vi "Initialise.vi"(8 "error in (no error)":errorcluster, 10 "Message in":refnum<class "InitialiseMessage.lvclass">, 11 "StageSPIM in":refnum<class "StageSPIM.lvclass">) -> (0 "error out":errorcluster, 3 "StageSPIM out":refnum<class "StageSPIM.lvclass">)   [LabVIEW 2012, in "StageSPIM.lvclass"]
doc: "This method is called when an initialise message is received. It mainly initialises the RabbitMQ connectivity. \n\nOverride this method when your component needs special initialisation (e.g. of software or hardware resources). In that case, don't forget to call the parent for proper implementation. If your component owns subcomponents, they count as resources, so you have to initialise them by calling their own initialise functions"
uses:
  StageSPIM.lvclass
  <vilib>/Distrio/Murmex/InitialiseMessage/InitialiseMessage.lvclass
  <vilib>/Distrio/Murmex/Murmex/Murmex.lvclass
  StageSPIM.lvclass/StageSPIM.ctl
panel:
  # "This method is called when the INTIALISE\ntrigger is sent. \n\nOverride this method when your component needs to\nrespond to this trigger. \n\nCall parent for proper implementation"
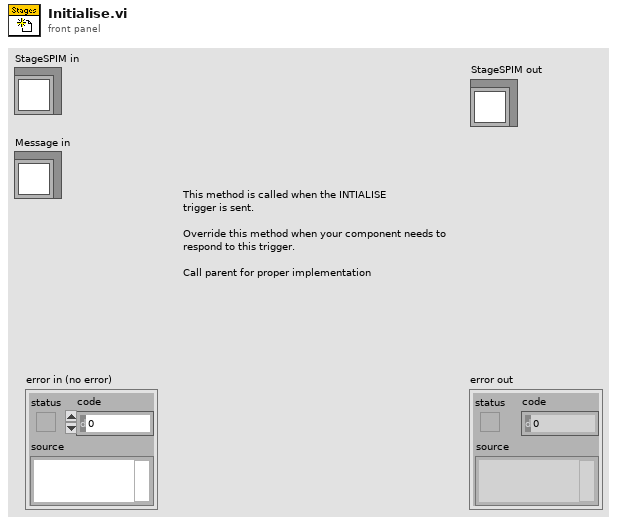
[diagram p1: front panel]
types:
  T1 = cluster{"Register DC":bool, "DaisyChain Search?":bool, "Device ID":i32}[][]
  T2 = cluster{"RON Affected axes":string[], "Reference mode":bool[], "Check FRF?":bool}
  T3 = typedef "StageSPIM.lvclass/port_control.ctl" = i32
  T4 = typedef "StageSPIM.lvclass/baud_rate_control.ctl" = u16
  T5 = typedef "StageSPIM.lvclass/connection_type.ctl" = enum16{"RS232", "RS232 DaisyChain", "USB", "USB_DaisyChain"}
  T6 = cluster{"Register DC":bool, "DaisyChain Search?":bool, "Device ID":i32}
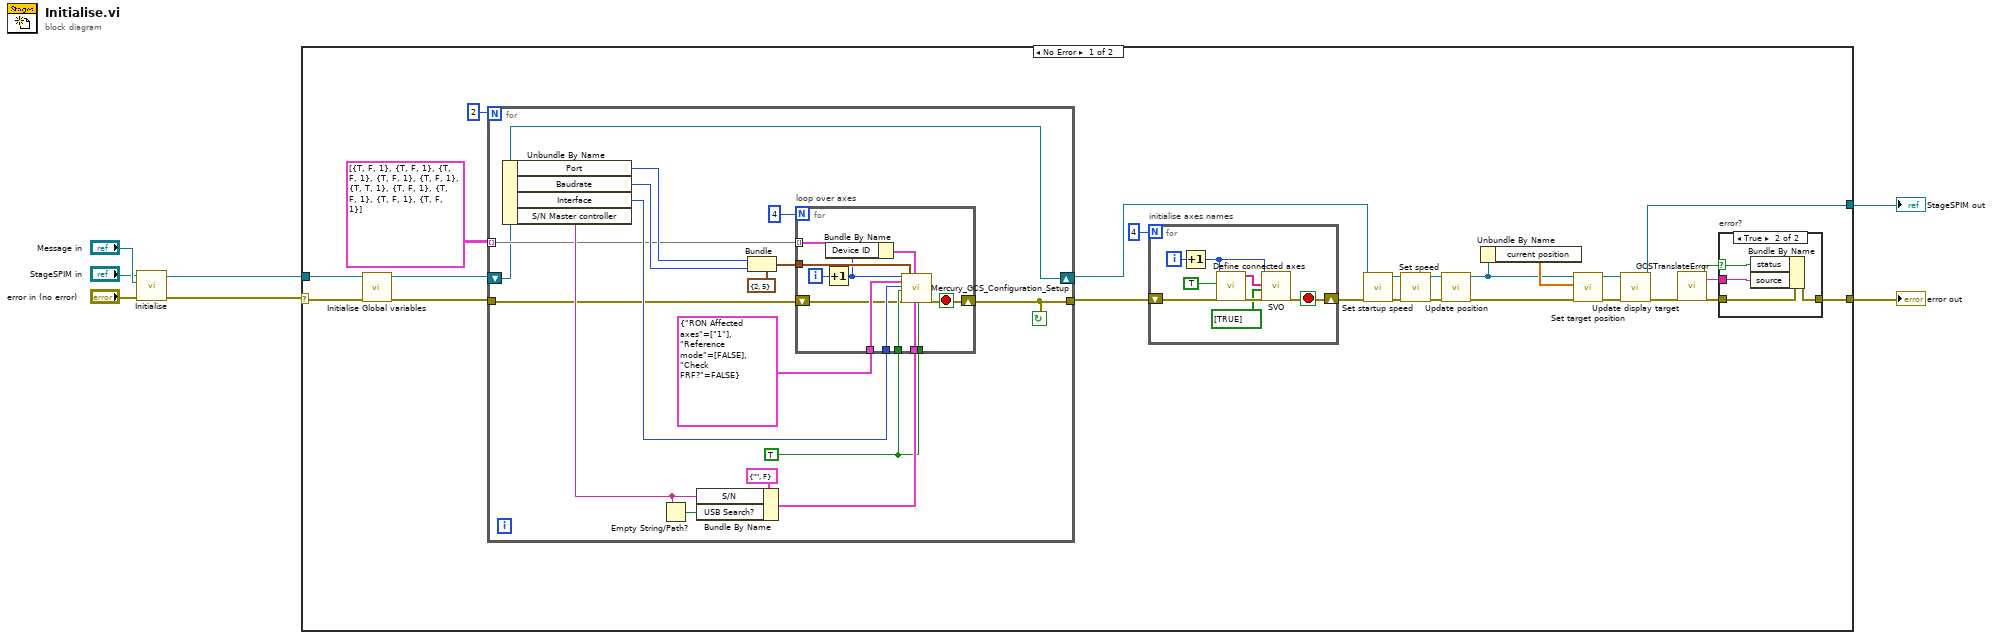
[diagram p0: block diagram]
diagram:
  n1 = call-parent "Initialise.vi"("error in (no error)"="error in (no error)", "Message in"="Message in", "Murmex in"="StageSPIM in") -> ("error out"=w4:errorcluster, "Murmex out"=w3:refnum<class "StageSPIM.lvclass">)  [unwired: 7 in]
  n2 = case shown="No Error" w4 {
    selector: w4 -> [w23 w75]
    tunnel: w3 -> [w21 w74]
    tunnel: [w12 w74] -> w2
    tunnel: [w24 w75] -> w1
    frame No Error {
      n3 = call-dynamic "Initialise Global variables.vi"("error in (no error)"=w23, "StageSPIM in"=w21) -> ("error out"=w22:errorcluster, "StageSPIM out"=w20:refnum<class "StageSPIM.lvclass">)  [unwired: 8 in]
      n4 = for {
        N: 2 -> [_]
        tunnel: [w34] -> w27
        tunnel: w22 -> [w37]
        tunnel: T1 [[{"Register DC"=TRUE, "DaisyChain Search?"=FALSE, "Device ID"=1}, {"Register DC"=TRUE, "DaisyChain Search?"=FALSE, "Device ID"=1}, {"Register DC"=TRUE, "DaisyChain Search?"=FALSE, "Device ID"=1}, {"Register DC"=TRUE, "DaisyChain Search?"=FALSE, "Device ID"=1}, {"Register DC"=TRUE, "DaisyChain Search?"=FALSE, "Device ID"=1}], [{"Register DC"=TRUE, "DaisyChain Search?"=TRUE, "Device ID"=1}, {"Register DC"=TRUE, "DaisyChain Search?"=FALSE, "Device ID"=1}, {"Register DC"=TRUE, "DaisyChain Search?"=FALSE, "Device ID"=1}, {"Register DC"=TRUE, "DaisyChain Search?"=FALSE, "Device ID"=1}, {"Register DC"=TRUE, "DaisyChain Search?"=FALSE, "Device ID"=1}]] -> [w36] mode=indexing
        shift-right: [w35] -> w9
        shift-left: w20 -> [w35]
        stop <- w34 continue-if-true
        w42 = TRUE ("Switch servo on?")
        n5 = Unbundle By Name(w35) -> ("Port"=w40:T3, "Baudrate"=w39:T4, "Interface"=w38:T5, "S/N Master controller"=w44:string)
        n6 = Empty String/Path?(string/path=w44) -> (empty?=w45:bool)
        n7 = Bundle By Name(cluster=cluster{"S/N":string, "USB Search?":bool} {"S/N"="", "USB Search?"=FALSE} ("USB settings"), "S/N"=w44, "USB Search?"=w45) -> (w43:cluster{"S/N":string, "USB Search?":bool})
        n8 = Bundle(cluster=cluster{"Portnumber":i32, "Baudrate":u16} {"Portnumber"=2, "Baudrate"=5} ("RS232 settings"), "Portnumber"=w40, "Baudrate"=w39) -> (w47:cluster{"Portnumber":i32, "Baudrate":u16})
        n9 = for "loop over axes" {
          N: 4 -> [_]
          tunnel: w36 -> [w53] mode=indexing
          tunnel: w38 -> [w60]
          tunnel: w42 -> [w55]
          tunnel: w47 -> [w59]
          tunnel: T2 {"RON Affected axes"=["1"], "Reference mode"=[FALSE], "Check FRF?"=FALSE} ("RON settings") -> [w58]
          tunnel: w43 -> [w57]
          shift-right: [w56] -> w34
          shift-left: w37 -> [w50]
          tunnel: w42 -> [w54]
          i -> [w49]
          stop <- w56 stop-if-true
          n10 = Increment(x=w49) -> (x+1=w51:i32)
          n11 = Bundle By Name(cluster=w53, "Device ID"=w51) -> (w52:T6)
          n12 = call "Mercury_GCS_Configuration_Setup.vi"("System no."=w51, "RON settings"=w58, "Interface"=w60, "All axes?"=w54, "error in"=w50, "RS232 settings"=w59, "DaisyChain settings"=w52, "USB settings"=w57, "Switch servo on?"=w55) -> ("error out"=w56:errorcluster)  [unwired: 4 in, 6 out]
        }
      }
      n13 = for "initialise axes names" {
        N: 4 -> [_]
        shift-right: [w66] -> w11
        shift-left: w27 -> [w73]
        i -> [w71]
        stop <- w66 stop-if-true
        n14 = Increment(x=w71) -> (x+1=w67:i32)
        n15 = call "Define connected axes.vi"("System no."=w67, "Read from\ncontroller?"=TRUE ("Read from\ncontroller?"), "error in"=w73) -> ("Conn. Axes out"=w68:string[], "error out"=w70:errorcluster)  [unwired: 15 in]
        n16 = call "SVO.vi"("System no."=w67, "Axes to command"=w68, "Servo mode"=bool[] [TRUE], "error in"=w70) -> ("error out"=w66:errorcluster)  [unwired: 15 in]
      }
      n17 = call-dynamic "Set startup speed.vi"("error in (no error)"=w11, "StageSPIM in"=w9) -> ("error out"=w10:errorcluster, "StageSPIM out"=w8:refnum<class "StageSPIM.lvclass">)  [unwired: 8 in]
      n18 = call-dynamic "Set speed.vi"("error in (no error)"=w10, "StageSPIM in"=w8) -> ("error out"=w25:errorcluster, "StageSPIM out"=w18:refnum<class "StageSPIM.lvclass">)  [unwired: 8 in]
      n19 = call-dynamic "Update position.vi"("error in (no error)"=w25, "StageSPIM in"=w18) -> ("error out"=w19:errorcluster, "StageSPIM out"=w14:refnum<class "StageSPIM.lvclass">)  [unwired: 8 in]
      n20 = Unbundle By Name(w14) -> ("current position"=w15:dbl[])
      n21 = call-dynamic "Set target position.vi"("error in (no error)"=w19, "target position"=w15, "StageSPIM in"=w14) -> ("error out"=w17:errorcluster, "StageSPIM out"=w13:refnum<class "StageSPIM.lvclass">)  [unwired: 7 in]
      n22 = call-dynamic "Update display target.vi"("error in (no error)"=w17, "StageSPIM in"=w13) -> ("error out"=w16:errorcluster, "StageSPIM out"=w12:refnum<class "StageSPIM.lvclass">)  [unwired: 8 in]
      n23 = call "GCSTranslateError.vi"("error in"=w16) -> ("GCS Error?"=w32:bool, "Error Description"=w30:string, "error out"=w31:errorcluster)  [unwired: 16 in]
      n24 = case "error?" shown="True" w32 {
        selector: w32 -> [_ w64]
        tunnel: w31 -> [w61 w65]
        tunnel: w30 -> [_ w63]
        tunnel: [w61 w62] -> w24
        frame False {
        }
        frame True {
          n25 = Bundle By Name(cluster=w65, "status"=w64, "source"=w63) -> (w62:errorcluster)
        }
      }
    }
    frame Error {
    }
  }
  "error out" <- w1
  "StageSPIM out" <- w2
